vi "Test CONNECT packet.vi"(8 "error in (no error)":errorcluster) -> (0 "error out":errorcluster)   [LabVIEW 2013]
uses:
  source/Control Packets/CONNECT/CONNECT.lvclass
  source/Control Packets/CONNECT/ConnectFlags -- cluster.ctl
  source/Control Packets/CONNECT/ConnectPayload -- cluster.ctl
  <vilib>/addons/_JKI Toolkits/Caraya/classes/Assert/Assert Equal Value_Variant.vi
  <vilib>/addons/_JKI Toolkits/Caraya/classes/Test/Test.lvclass
  <vilib>/addons/_JKI Toolkits/Caraya/classes/Assert/Assert.lvclass
  source/Control Packets/ControlPacket/ControlPacket.lvclass
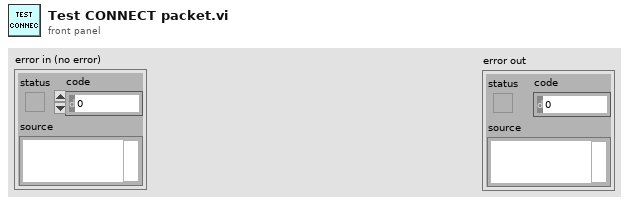
[diagram p1: front panel]
types:
  T1 = typedef "MQTT_Control_Packets.lvlib/CONNECT.lvclass/ConnectPayload -- cluster.ctl" = cluster{"Will Topic":string, "Will Message":string, "Username":string, "Password":string}
  T2 = typedef "MQTT_Control_Packets.lvlib/CONNECT.lvclass/ConnectFlags -- cluster.ctl" = cluster{"Reserved":bool, "Clean Session":bool, "Will Flag":bool, "Will QoS 1":bool, "Will QoS 2":bool, "Will Retain":bool, "Password Flag":bool, "User Name Flag":bool}
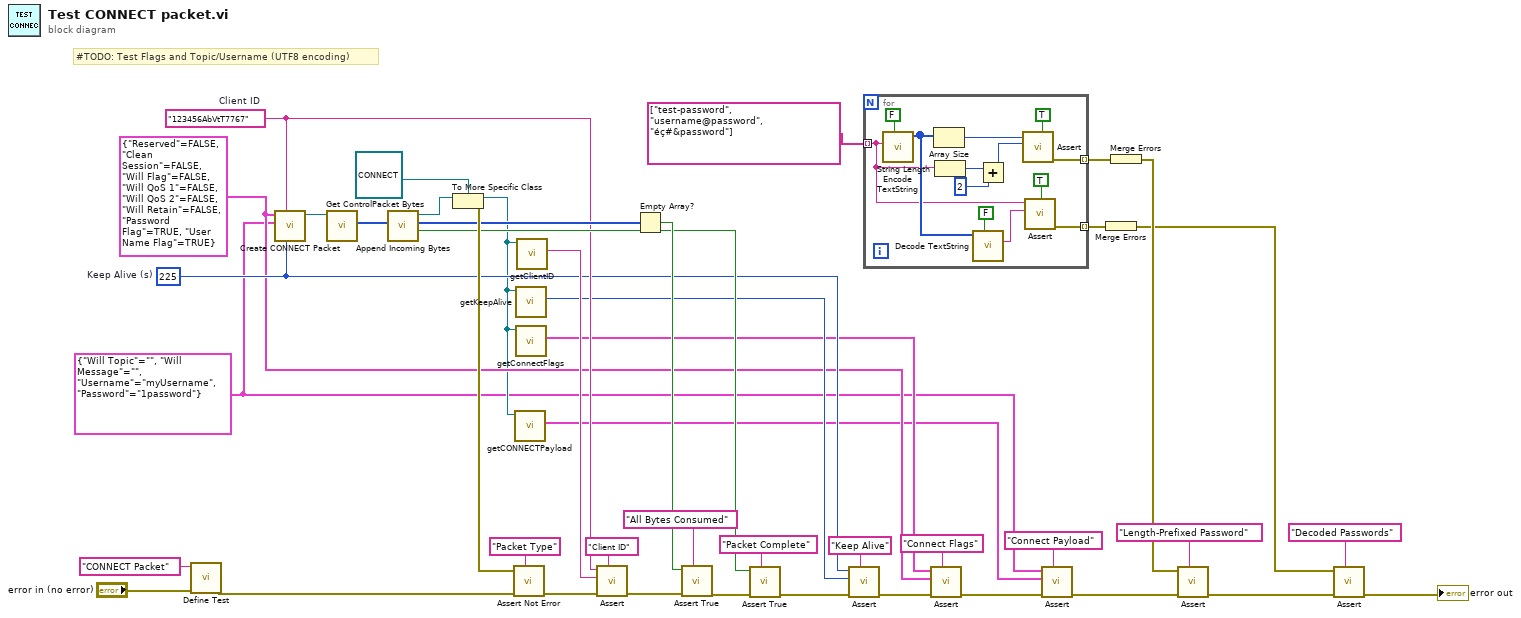
[diagram p0: block diagram]
diagram:
  w3 = T1 {"Will Topic"="", "Will Message"="", "Username"="myUsername", "Password"="1password"} ("Payload")
  w18 = T2 {"Reserved"=FALSE, "Clean Session"=FALSE, "Will Flag"=FALSE, "Will QoS 1"=FALSE, "Will QoS 2"=FALSE, "Will Retain"=FALSE, "Password Flag"=TRUE, "User Name Flag"=TRUE} ("Connect Flags")
  w22 = u16 225  # Keep Alive (s)
  w28 = "123456AbVtT7767"  # Client ID
  # "#TODO: Test Flags and Topic/Username (UTF8 encoding)"
  n1 = call <vilib>:"Define Test.vi"("error in (no error)"="error in (no error)", "Label (VI Title)"="CONNECT Packet") -> ("error out"=w41:errorcluster)  [unwired: 9 in]
  n2 = call "Create CONNECT Packet.vi"("Keep Alive (s)"=w22, "Client ID (empty: generate new)"=w28, "Payload"=w3, "Connect Flags"=w18) -> ("CONNECT"=w33:refnum<class "CONNECT.lvclass">)  [unwired: 5 in, 2 out]
  n3 = call "Get ControlPacket Bytes.vi"("ControlPacket"=w33) -> ("Bytes Stream"=w32:u8[])  [unwired: 7 in, 3 out]
  n4 = call "Append Incoming Bytes.vi"("Incoming Packets"=w32) -> ("Complete Packet"=w29:bool, "Remaining Packets"=w30:u8[], "ControlPacket"=w31:refnum<class "ControlPacket.lvclass">)  [unwired: 7 in, 1 out]
  n5 = To More Specific Class(target class=refnum<class "CONNECT.lvclass"> refnum ("MQTT_Control_Packets.lvlib:CONNECT.lvclass"), reference=w31) -> (specific class reference=w6:refnum<class "CONNECT.lvclass">, error out=w40:errorcluster)  [unwired: 1 in]
  n6 = call <vilib>:"Assert Not Error.vi"("Label"="Packet Type" ("Label (VI Title)"), "error in (no error)"=w41, "Not Error?"=w40) -> ("error out"=w26:errorcluster)  [unwired: 8 in]
  n7 = call "getCONNECTPayload.vi"("CONNECT in"=w6) -> ("Payload"=w2:T1)  [unwired: 9 in, 1 out]
  n8 = call "getKeepAlive.vi"("CONNECT in"=w6) -> ("Keep Alive (s)"=w21:u16)  [unwired: 9 in, 1 out]
  n9 = call "getConnectFlags.vi"("CONNECT in"=w6) -> ("Connect Flags"=w19:T2)  [unwired: 9 in, 1 out]
  n10 = call "getClientID.vi"("CONNECT in"=w6) -> ("Client ID"=w27:string)  [unwired: 9 in, 1 out]
  n11 = call-poly <vilib>:"Assert.vi"("Label"="Client ID" ("Label (VI Title)"), "error in (no error)"=w26, "Y"=w27, "X"=w28) -> ("error out"=w25:errorcluster)  [unwired: 7 in]
  n12 = Empty Array?(array=w30) -> (empty?=w38:bool)
  n13 = call <vilib>:"Assert True.vi"("Label"="All Bytes Consumed" ("Label (VI Title)"), "error in (no error)"=w25, "True?"=w38) -> ("error out"=w36:errorcluster)  [unwired: 8 in]
  n14 = call <vilib>:"Assert True.vi"("Label"="Packet Complete" ("Label (VI Title)"), "error in (no error)"=w36, "True?"=w29) -> ("error out"=w20:errorcluster)  [unwired: 8 in]
  n15 = call-poly <vilib>:"Assert.vi"("Label"="Keep Alive" ("Label (VI Title)"), "error in (no error)"=w20, "Y"=w21, "X"=w22) -> ("error out"=w17:errorcluster)  [unwired: 7 in]
  n16 = for {
    tunnel: string[] ["test-password", "username@password", "éç#&password"] -> [w46] mode=indexing
    tunnel: [w50] -> w13 mode=indexing
    tunnel: [w45] -> w8 mode=indexing
    n17 = call "Encode TextString.vi"("Convert to UTF8? (T)"=FALSE, "Text String"=w46) -> ("Length-Prefixed Field"=w48:u8[])  [unwired: 9 in]
    n18 = Array Size(array=w48) -> (size(s)=w53:i32)
    n19 = String Length(string=w46) -> (length=w55:i32)
    n20 = call "Decode TextString.vi"("Decode from UTF8? (T)"=FALSE ("Convert to UTF8? (T)"), "Length-Prefixed Field"=w48) -> ("Text String"=w47:string)  [unwired: 7 in, 2 out]
    n21 = Add(x=w55, y=2) -> (x+y=w52:i32)
    n22 = call-poly <vilib>:"Assert.vi"("Assert Only? (F)"=TRUE, "Y"=w52, "X"=w53) -> ("error out"=w50:errorcluster)  [unwired: 8 in]
    n23 = call-poly <vilib>:"Assert.vi"("Assert Only? (F)"=TRUE, "Y"=w47, "X"=w46) -> ("error out"=w45:errorcluster)  [unwired: 8 in]
  }
  n24 = call-poly <vilib>:"Assert.vi"("Label"="Connect Flags" ("Label (VI Title)"), "error in (no error)"=w17, "Y"=w18, "X"=w19) -> ("error out"=w5:errorcluster)  [unwired: 7 in]
  n25 = call-poly <vilib>:"Assert.vi"("Label"="Connect Payload" ("Label (VI Title)"), "error in (no error)"=w5, "Y"=w2, "X"=w3) -> ("error out"=w4:errorcluster)  [unwired: 7 in]
  n26 = Merge Errors(w8) -> (w7:errorcluster)
  n27 = Merge Errors(w13) -> (w12:errorcluster)
  n28 = call-poly <vilib>:"Assert.vi"("Label"="Length-Prefixed Password" ("Label (VI Title)"), "error in (no error)"=w4, "Not Error?"=w12) -> ("error out"=w10:errorcluster)  [unwired: 8 in]
  n29 = call-poly <vilib>:"Assert.vi"("Label"="Decoded Passwords" ("Label (VI Title)"), "error in (no error)"=w10, "Not Error?"=w7) -> ("error out"=→"error out":errorcluster)  [unwired: 8 in]
